vi "Com_Matrix220_Parse Message.vi"(8 "error in":errorcluster, 10 "Message Type":T1=enum."Code", 11 "Message":string) -> (0 "error out":errorcluster, 3 "Variant":variant)   [LabVIEW 2016]
uses:
  Data Def/Com_Matrix220_Message Type.ctl
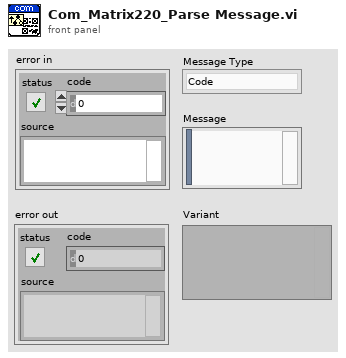
[diagram p1: front panel]
types:
  T1 = typedef "Com_Matrix220_Message Type.ctl" = enum16{"Unkown", "Ack", "Code", "Image"}
  T2 = typedef "imagedata.ctl" = cluster{"image type":i32, "image depth":i32, "image":u8[], "mask":u8[], "colors":u32[], "Rectangle":cluster{"left":i16, "top":i16, "right":i16, "bottom":i16}}
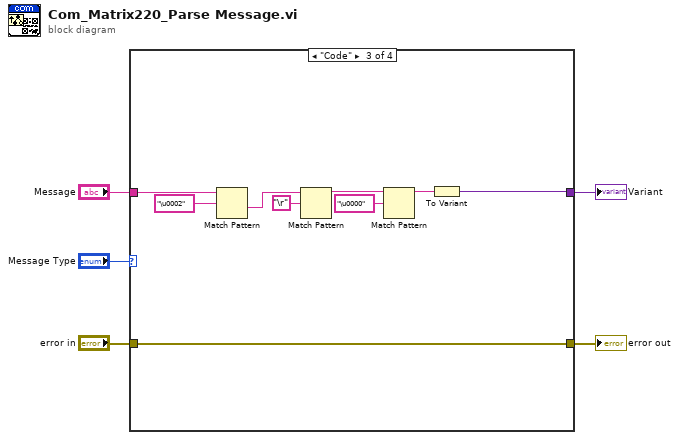
[diagram p0: block diagram]
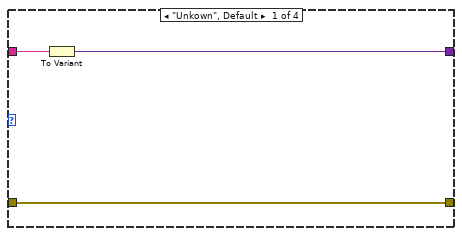
[diagram p2: hidden frame]
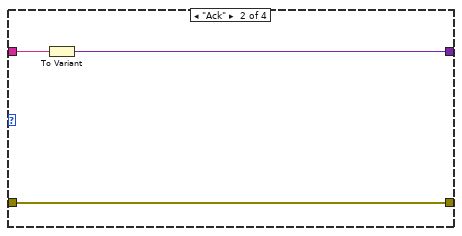
[diagram p3: hidden frame]
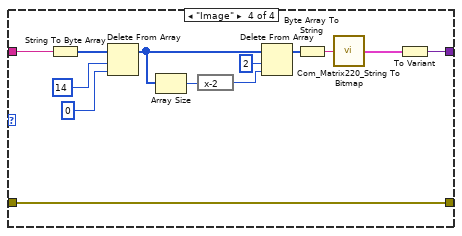
[diagram p4: hidden frame]
diagram:
  n1 = case shown="\"Code\"" "Message Type" {
    tunnel: "Message" -> [w8 w11 w18 w33]
    tunnel: "error in" -> [w6 w9 w19 w21]
    tunnel: [w7 w10 w20 w22] -> w2
    tunnel: [w6 w9 w19 w21] -> w1
    frame "Unkown", Default {
      n2 = To Variant(anything=w8) -> (Variant=w7:variant)
    }
    frame "Ack" {
      n3 = To Variant(anything=w11) -> (Variant=w10:variant)
    }
    frame "Code" {
      n4 = Match Pattern(string=w18, regular expression="\u0002") -> (after substring=w16:string)  [unwired: 1 in, 3 out]
      n5 = Match Pattern(string=w16, regular expression="\r") -> (before substring=w14:string)  [unwired: 1 in, 3 out]
      n6 = Match Pattern(string=w14, regular expression="\u0000") -> (before substring=w13:string)  [unwired: 1 in, 3 out]
      n7 = To Variant(anything=w13) -> (Variant=w20:variant)
    }
    frame "Image" {
      n8 = String To Byte Array(string=w33) -> (unsigned byte array=w32:u8[])
      n9 = Delete From Array(array=w32, length=14, index=0) -> (array with subset deleted=w25:u8[])  [unwired: 1 out]
      n10 = Array Size(array=w25) -> (size(s)=w29:i32)
      n11 = expression code="x-2"(w29) -> (w28:i32)
      n12 = Delete From Array(array=w25, length=2, index=w28) -> (array with subset deleted=w26:u8[])  [unwired: 1 out]
      n13 = Byte Array To String(unsigned byte array=w26) -> (string=w24:string)
      n14 = call "Com_Matrix220_String To Bitmap.vi"("String"=w24) -> ("Image Data"=w23:T2)  [unwired: 2 in, 1 out]
      n15 = To Variant(anything=w23) -> (Variant=w22:variant)
    }
  }
  "error out" <- w1
  "Variant" <- w2
